vi "Handshake.vi"(8 "error in (no error)":errorcluster, 9 "Timeout (5000ms)":i32=5000, 11 "dotNET SSL Client Socket in":refnum<class "dotNET SSL Client Socket.lvclass">) -> (0 "error out":errorcluster, 3 "dotNET SSL Client Socket out":refnum<class "dotNET SSL Client Socket.lvclass">)   [LabVIEW 2013, in "dotNET SSL Socket.lvlib" / "dotNET SSL Client Socket.lvclass"]
uses:
  dotNET SSL Client Socket.lvclass
  dotNET SSL Socket/dotNET SSL Socket.lvclass/dotNET SSL Socket.ctl
  dotNET SSL Client Socket.lvclass/dotNET SSL Client Socket.ctl
  dotNET SSL Socket/Read SSLStream.vi
  Read Hostname _ URL.vi
  Read clientCertificates.vi
  dotNET SSL Socket/Read Check Revocation.vi
  dotNET SSL Socket/Read Masked SSL Protocols.vi
  <vilib>/MediaMongrels Ltd/WebSockets/WebSockets/WebSocket Client/WebSocket Client.lvclass
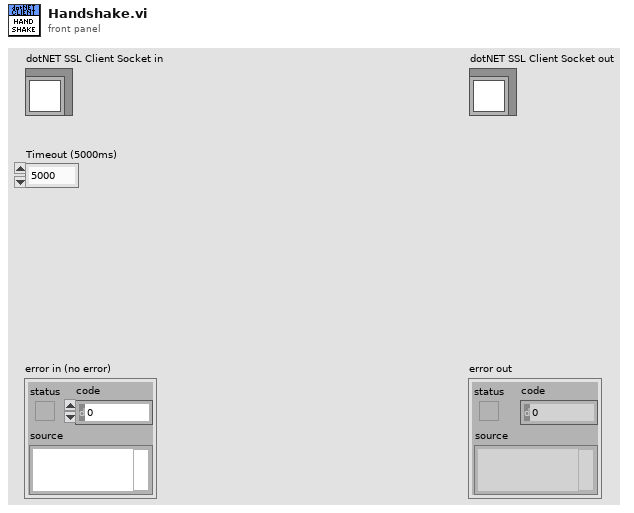
[diagram p1: front panel]
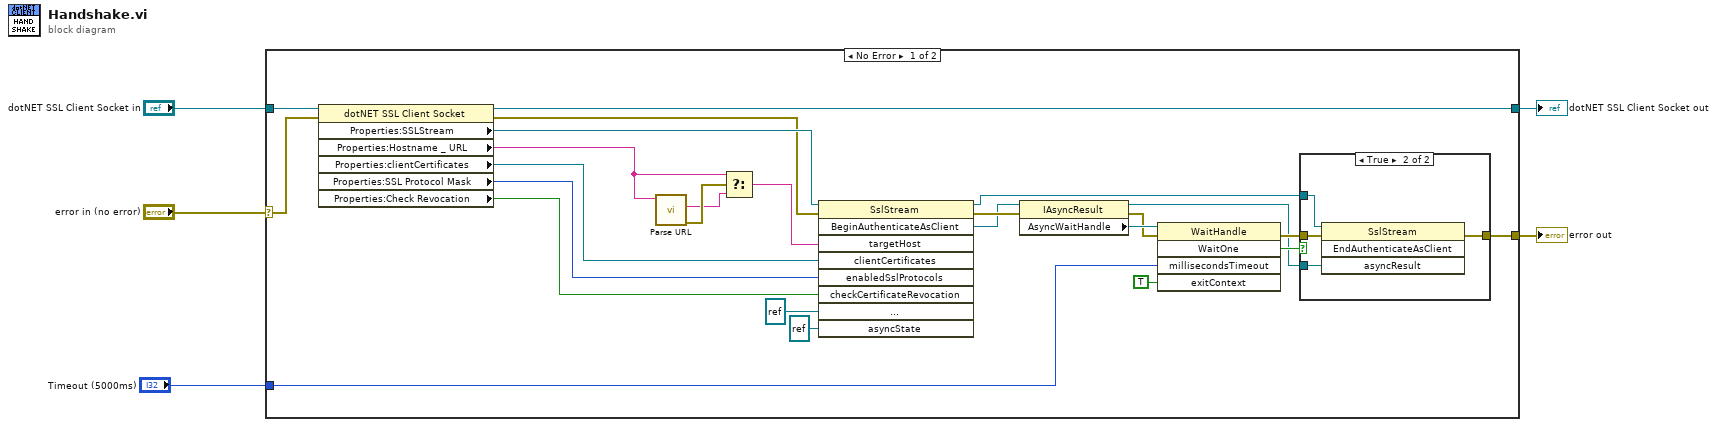
[diagram p0: block diagram]
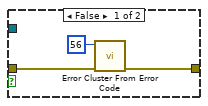
[diagram p2: hidden frame]
diagram:
  n1 = case shown="No Error" "error in (no error)" {
    selector: "error in (no error)" -> [w19 w39]
    tunnel: [w18 w39] -> w4
    tunnel: [w20 w38] -> w2
    tunnel: "dotNET SSL Client Socket in" -> [w30 w38]
    tunnel: "Timeout (5000ms)" -> [w15 _]
    frame No Error {
      n2 = property class="dotNET SSL Client Socket"(reference=w30, error in=w19) -> (reference out=w20:refnum<class "dotNET SSL Client Socket.lvclass">, error out=w16:errorcluster, "Properties:SSLStream"=w17:refnum<k24>, "Properties:Hostname _ URL"=w13:string, "Properties:clientCertificates"=w7:refnum<k24>, "Properties:SSL Protocol Mask"=w8:i32, "Properties:Check Revocation"=w6:bool)
      n3 = call <vilib>:"Parse URL.vi"("WebSocket URL"=w13) -> ("error out"=w14:errorcluster, "host"=w11:string)  [unwired: 6 in, 3 out]
      n4 = Select(t=w13, s=w14, f=w11) -> (s? t:f=w12:string)
      n5 = invoke class="SslStream" method="BeginAuthenticateAsClient"(reference=w17, error in=w16, "targetHost"=w12, "clientCertificates"=w7, "enabledSslProtocols"=w8, "checkCertificateRevocation"=w6, "asyncCallback"=refnum<k24> refnum, "asyncState"=refnum<k24> refnum) -> (reference out=w21:refnum<k24>, error out=w29:errorcluster, "BeginAuthenticateAsClient"=w28:refnum<k24>)  [unwired: 1 in, 6 out]
      n6 = property class="IAsyncResult"(reference=w28, error in=w29) -> (reference out=w22:refnum<k24>, error out=w26:errorcluster, "AsyncWaitHandle"=w27:refnum<k24>)
      n7 = invoke class="WaitHandle" method="WaitOne"(reference=w27, error in=w26, "millisecondsTimeout"=w15, "exitContext"=TRUE) -> (error out=w23:errorcluster, "WaitOne"=w24:bool)  [unwired: 1 in, 3 out]
      n8 = case shown="True" w24 {
        tunnel: w23 -> [w32 w37]
        tunnel: [w31 w35] -> w18
        tunnel: w22 -> [_ w36]
        tunnel: w21 -> [_ w34]
        frame False {
          n9 = call <vilib>:"Error Cluster From Error Code.vi"("error in (no error)"=w32, "error code (0)"=56) -> ("error out"=w31:errorcluster)  [unwired: 7 in]
        }
        frame True {
          n10 = invoke class="SslStream" method="EndAuthenticateAsClient"(reference=w34, error in=w37, "asyncResult"=w36) -> (error out=w35:errorcluster)  [unwired: 1 in, 3 out]
        }
      }
    }
    frame Error {
    }
  }
  "error out" <- w4
  "dotNET SSL Client Socket out" <- w2
